vi "Configure Pulse.vi"(4 "Width (10 msec)":dbl=0.01 format="%.6p", 6 "Delay (10 msec)":dbl=0.01 format="%.6p", 7 "Channel (1:Chan A)":i32(ring)=1 items=["Channel A"=1, "Channel B"=2, "Channel C"=3, "Channel D"=4, "Channel E"=5, "Channel F"=6, "Channel G"=7, "Channel H"=8], 8 "error in (no error)":errorcluster, 9 "Wait # (0)":i32, 11 "VISA resource name":refnum<visa-resource-name>) -> (0 "error out":errorcluster, 3 "VISA resource name out":refnum<visa-resource-name>)   [LabVIEW 2020, in "Berkeley Nucleonics 500 Series.lvlib"]
doc: "This VI is used to configure the pulse timing for a channel."
uses:
  Berkeley Nucleonics 500 Series.lvlib
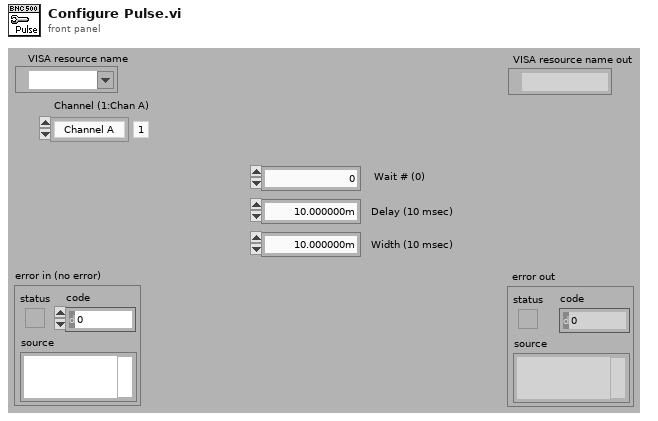
[diagram p1: front panel]
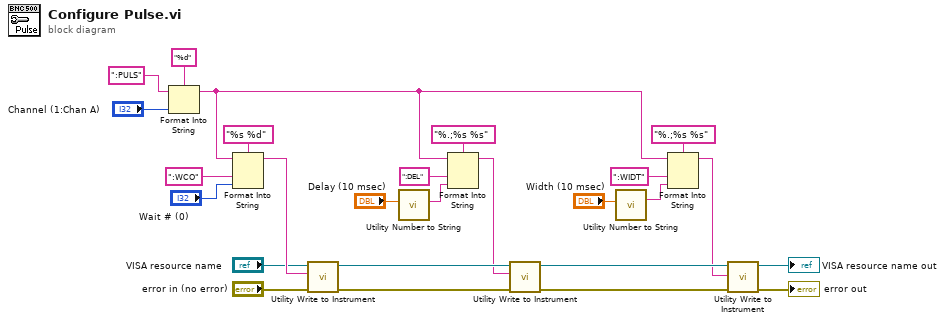
[diagram p0: block diagram]
diagram:
  n1 = Format Into String(format string="%d", initial string=":PULS", "Channel (1:Chan A)") -> (resulting string=w1:string)  [unwired: 1 in, 1 out]
  n2 = Format Into String(format string="%s %d", initial string=w1, ":WCO", "Wait # (0)") -> (resulting string=w12:string)  [unwired: 1 in, 1 out]
  n3 = call "Utility Write to Instrument.vi"("error in (no error)"="error in (no error)", "Write Buffer"=w12, "VISA resource name"="VISA resource name") -> ("error out"=w13:errorcluster, "VISA resource name out"=w14:refnum<visa-resource-name>)  [unwired: 6 in, 1 out]
  n4 = call "Utility Number to String.vi"("Numeric"="Delay (10 msec)") -> ("Shortest String"=w7:string)  [unwired: 10 in]
  n5 = Format Into String(format string="%.;%s %s", initial string=w1, ":DEL", w7) -> (resulting string=w6:string)  [unwired: 1 in, 1 out]
  n6 = call "Utility Write to Instrument.vi"("error in (no error)"=w13, "Write Buffer"=w6, "VISA resource name"=w14) -> ("error out"=w22:errorcluster, "VISA resource name out"=w23:refnum<visa-resource-name>)  [unwired: 6 in, 1 out]
  n7 = call "Utility Number to String.vi"("Numeric"="Width (10 msec)") -> ("Shortest String"=w5:string)  [unwired: 10 in]
  n8 = Format Into String(format string="%.;%s %s", initial string=w1, ":WIDT", w5) -> (resulting string=w3:string)  [unwired: 1 in, 1 out]
  n9 = call "Utility Write to Instrument.vi"("error in (no error)"=w22, "Write Buffer"=w3, "VISA resource name"=w23) -> ("error out"=→"error out":errorcluster, "VISA resource name out"=→"VISA resource name out":refnum<visa-resource-name>)  [unwired: 6 in, 1 out]
